vi "SICK Only.vi"() -> ()   [LabVIEW 2009]
uses:
  FPGA/SICK VI's/SICK Reader States.ctl
  Init State.ctl
  <vilib>/LabVIEW Targets/FPGA/cRIO/shared/nicrio_ModuleControls/nicrio_cRIO-9871_FlowControlEnum.ctl
  <vilib>/LabVIEW Targets/FPGA/cRIO/shared/nicrio_ModuleControls/nicrio_cRIO-9871_ParityEnum.ctl
  <vilib>/LabVIEW Targets/FPGA/cRIO/shared/nicrio_ModuleControls/nicrio_cRIO-9871_StopBitsEnum.ctl
  <vilib>/LabVIEW Targets/FPGA/cRIO/shared/nicrio_ModuleControls/nicrio_cRIO-9871_DataBitsEnum.ctl
  <vilib>/LabVIEW Targets/FPGA/cRIO/shared/nicrio_ModuleControls/nicrio_cRIO-9871_BaudRateEnum.ctl
  <vilib>/eio/EIOPropertyNode/EIOPropertyNode.xnode
  <vilib>/rvi/eio/nirviEIOPropertyImplementation/nirviEIOPropertyImplementation.xnode
  <vilib>/rvi/eio/common/nirviEmuTemplatePropertySet_errors.vi
  <vilib>/eio/EIOMethodNode/EIOMethodNode.xnode
  <vilib>/rvi/eio/nirviEIOMethodImplementation/nirviEIOMethodImplementation.xnode
  <vilib>/rvi/eio/common/nirviEmuTemplateMethod_errors.vi
  <vilib>/rvi/eio/common/nirviEmuClasses.ctl
  <vilib>/rvi/DataTransferAndStorage/Container/XNode/niFpgaContainer.xnode
  <vilib>/rvi/interface/RandomDataEmulation/niFpgaRandomDataHandleErrors.vi
  <vilib>/rvi/interface/RandomDataEmulation/nirviRandomDataFPGAFIFO.vi
  <vilib>/rvi/DataTransferAndStorage/Container/Common/niFpgaContainerMethod.ctl
  <vilib>/rvi/DataTransferAndStorage/Container/Common/niFpgaTransferTypeControl.ctl
  <vilib>/rvi/Memory/Memory_Emulation/nirvimemoryEmulationManagerCache_GetValue.vi
  <vilib>/rvi/Memory/Memory_Emulation/nirvimemoryEmulationManagerCache_InsertValue.vi
  <vilib>/rvi/FIFO/Fifo_Resource/nirvififoUniquifyingName.vi
  <vilib>/Utility/error.llb/Clear Errors.vi
  <vilib>/rvi/Memory/Memory_Emulation/nirvimemoryEmulationManagerCache_SetValue.vi
  <vilib>/rvi/eio/common/nirviEmuTemplatePropertyGet_errors.vi
panel:
  out "Responses Timeout":bool
  in  "Correct Response Timeout (ms)":i32=200
  out "SICK Init State":u8
  out "SICK Reader States":T1
  in  "EN mask overflow bytes":bool
  in  "En overflow replacement":bool
  out "Read Period":u32
  out "Tick count":u32
  out "Read data error":errorcluster
  in  "Read/Write Timeout (ms)":i32
  in  "Bytes at Port Timeout (us)":i32
  in  "Overflow Reading":u16
  out "No Data (timeout)":bool
  out "Initialization error":errorcluster
  out "RT commands timeout":bool
  out "Pre-initialization error":errorcluster
  out "Initialization success":bool
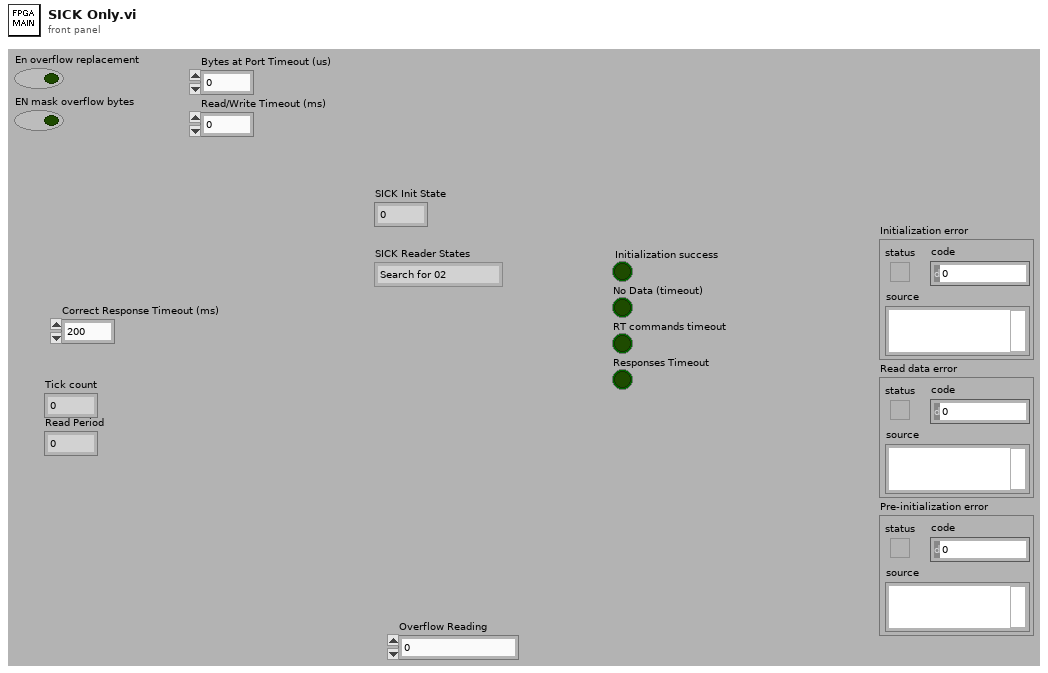
[diagram p1: front panel]
types:
  T1 = typedef "SICK Reader States.ctl" = enum16{"Search for 02", "Search for Header", "Read Data"}
  T2 = typedef "Init State.ctl" = u8
  T3 = typedef "nicrio_cRIO-9871_FlowControlEnum.ctl" = enum8{"None", "Software (XON / XOFF)", "Hardware (RTS / CTS)"}
  T4 = typedef "nicrio_cRIO-9871_ParityEnum.ctl" = enum8{"None", "Odd", "Even", "Mark", "Space"}
  T5 = typedef "nicrio_cRIO-9871_StopBitsEnum.ctl" = enum8{"1", "1.5", "2"}
  T6 = typedef "nicrio_cRIO-9871_DataBitsEnum.ctl" = enum8{"5", "6", "7", "8"}
  T7 = typedef "nicrio_cRIO-9871_BaudRateEnum.ctl" = enum16{"75 bps", "110 bps", "134 bps", "150 bps", "300 bps", "600 bps", "1200 bps", "1800 bps", "2400 bps", "4800 bps", "7200 bps", "9600 bps", "14.4 kbps", "19.2 kbps", "28.8 kbps", "38.4 kbps", "57.6 kbps", "115.2 kbps", "230.4 kbps", "460.8 kbps", "921.6 kbps"}
  T8 = typedef "nirviEmuClasses.ctl" = enum16{"IO Read", "IO Write", "Method", "Property Read", "Property Write"}
  T9 = typedef "niFpgaContainerMethod.ctl" = enum16{"Write", "Read", "Clear", "Get Number of Elements to Write", "Get Number of Elements to Read", "Enable", "Disable", "Flush and Disable", "Get Stream State"}
  T10 = typedef "niFpgaTransferTypeControl.ctl" = enum16{"Target-Scoped", "Host to Target - DMA", "Target to Host - DMA", "Peer to Peer Reader", "Peer to Peer Writer", "Bidirectional"}
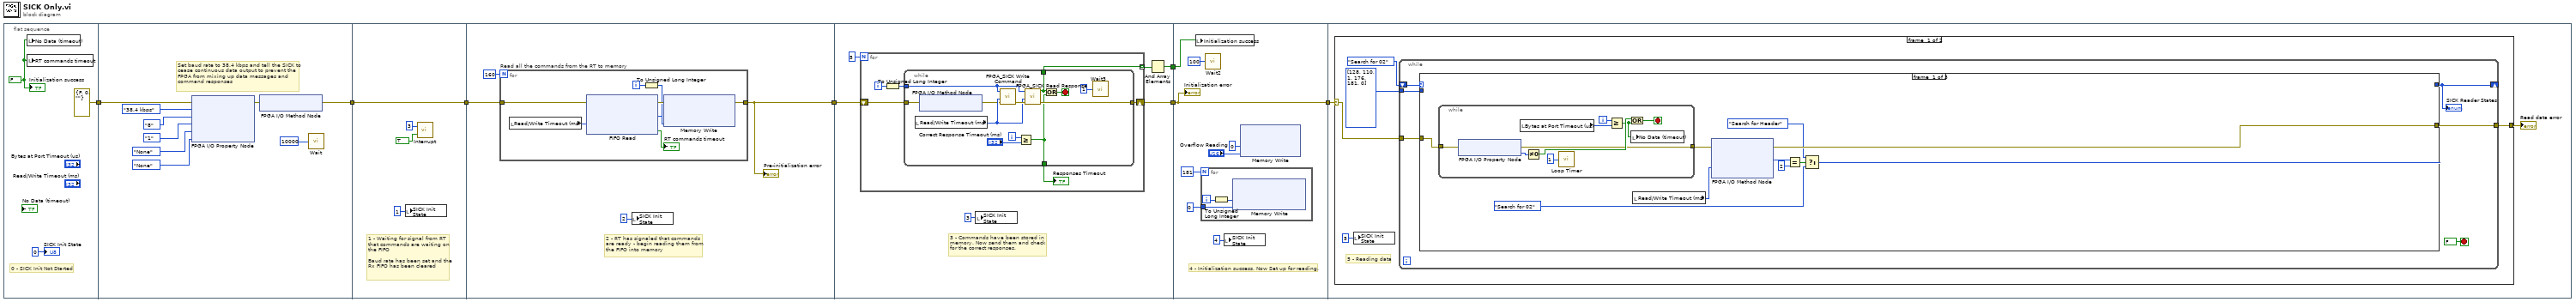
[diagram p0: block diagram]
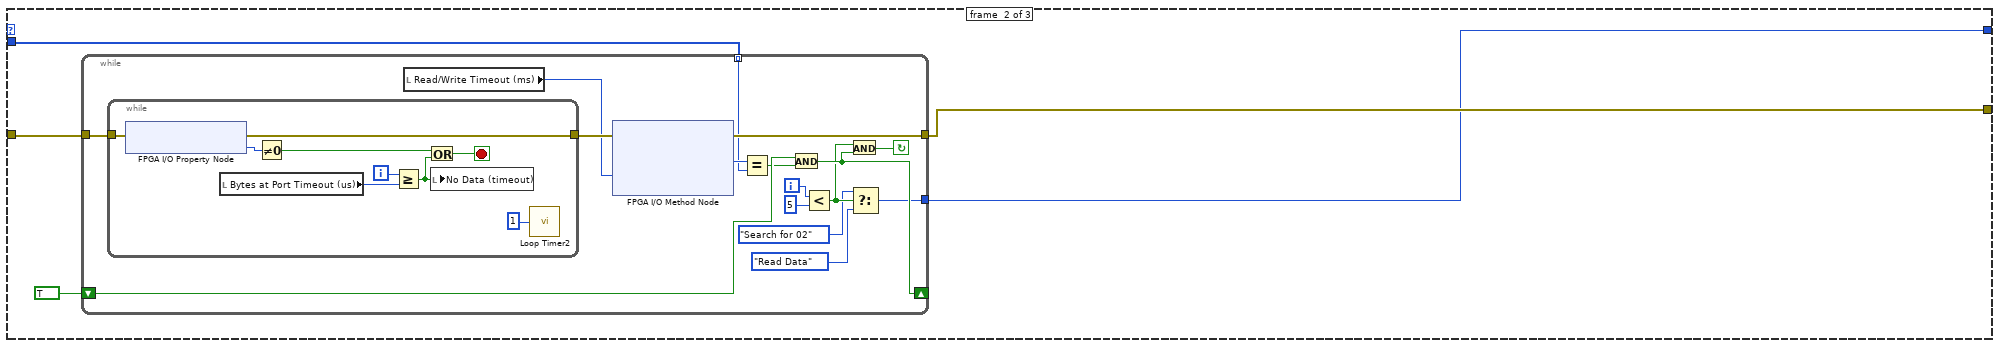
[diagram p2: hidden frame]
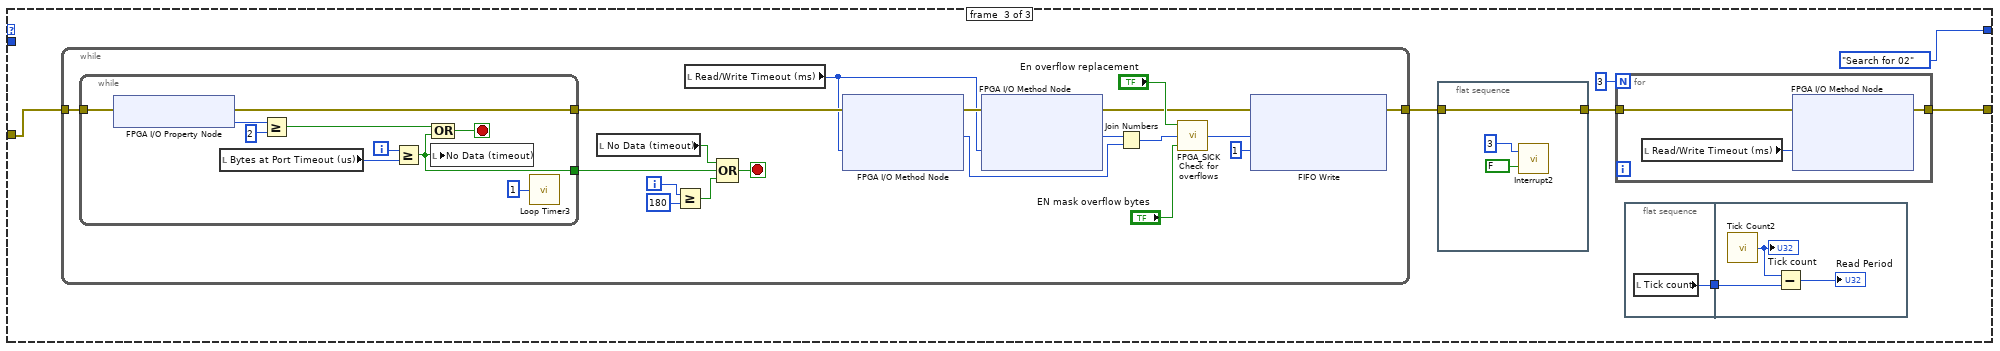
[diagram p3: hidden frame]
diagram:
  n1 = flat-sequence {
    tunnel: [errorcluster {"status"=FALSE, "code"=0, "source"=""} ("error out")] -> w6
    tunnel: w6 -> [w12]
    tunnel: [w11] -> w5
    tunnel: w5 -> [w78]
    tunnel: [w78] -> w4
    tunnel: w4 -> [w82]
    tunnel: [w80] -> w2
    tunnel: [w253] -> w3
    tunnel: w2 -> [w256]
    tunnel: [w252] -> w1
    tunnel: w3 -> [w287]
    tunnel: [w287] -> w7
    tunnel: w1 -> [w286]
    tunnel: w7 -> [w551]
    frame #0 {
      w10 = FALSE ("Initialization complete")
      # "0 - SICK Init Not Started"
      n2 = local write "No Data (timeout)"(w10) -> ()
      n3 = local write "RT commands timeout"(w10) -> ()
      "Initialization success" <- w10
      "SICK Init State" <- T2 0 ("SICK Init State")
    }
    frame #1 {
      # "Set baud rate to 38.4 kbps and tell the SICK to \ncease continuous data output to prevent the \nFPGA from mixing up data messages and \ncommand responses"
      n4 = xnode "FPGA I/O Property Node"("error in"=w12, "Baud Rate"=nicrio_cRIO-9871_BaudRateEnum."38.4 kbps", "Data Bits"=nicrio_cRIO-9871_DataBitsEnum."8", "Stop Bits"=nicrio_cRIO-9871_StopBitsEnum."1", "Parity"=nicrio_cRIO-9871_ParityEnum."None", "Flow Control"=nicrio_cRIO-9871_FlowControlEnum."None") -> ("error out"=w14:errorcluster)  [unwired: 1 in, 1 out]
      n5 = xnode "FPGA I/O Method Node"("error in"=w14) -> ("error out"=w11:errorcluster)  [unwired: 1 in, 1 out]
      n6 = call "Wait"("Count(uSec)"=u32 10000 ("Set new baud rate wait (usec)")) -> ()  [unwired: 1 out]
    }
    frame #2 {
      # "1 - Waiting for signal from RT\nthat commands are waiting on\nthe FIFO\n\nBaud rate has been set and the\nRx FIFO has been cleared"
      n7 = local write "SICK Init State"(T2 1 ("SICK Init State")) -> ()
      n8 = call "Interrupt"("Wait Until Cleared"=TRUE, "IRQ Number"=u8 3) -> ()  [unwired: 1 out]
    }
    frame #3 {
      # "2 - RT has signaled that commands\nare ready - begin reading them from\nthe FIFO into memory"
      n9 = for "Read all the commands from the RT to memory" {
        N: 160 -> [_]
        tunnel: [w89] -> w80
        tunnel: w82 -> [w84]
        i -> [w86]
        n10 = local read "Read/Write Timeout (ms)"() -> (w88:i32)
        n11 = xnode ("FIFO Read")("Timeout"=w88, "error in (no error)"=w84) -> ("Element"=w91:u8, "Timed Out?"=→"RT commands timeout":bool, "error out"=w90:errorcluster)  [unwired: 1 in, 1 out]
        n12 = To Unsigned Long Integer(number=w86) -> (unsigned 32bit integer=w85:u32)
        n13 = xnode ("Memory Write")("Address"=w85, "Data"=w91, "error in (no error)"=w90) -> ("error out"=w89:errorcluster)  [unwired: 1 in, 1 out]
      }
      "Pre-initialization error" <- w80
      n14 = local write "SICK Init State"(T2 2 ("SICK Init State")) -> ()
    }
    frame #4 {
      # "3 - Commands have been stored in\nmemory. Now send them and check\nfor the correct responses."
      n15 = for {
        N: 5 -> [_]
        shift-right: [w261] -> w253
        shift-left: w256 -> [w262]
        tunnel: [w258] -> w254 mode=indexing
        i -> [w260]
        n16 = To Unsigned Long Integer(number=w260) -> (unsigned 32bit integer=w259:u32)
        n17 = while {
          tunnel: w262 -> [w265]
          tunnel: [w274] -> w261
          tunnel: w259 -> [w271]
          tunnel: [w270] -> w258
          tunnel: [w263] -> w257
          i -> [w268]
          stop <- w266 stop-if-true
          n18 = local read "Read/Write Timeout (ms)"() -> (w272:i32)
          n19 = xnode "FPGA I/O Method Node"("error in"=w265) -> ("error out"=w264:errorcluster)  [unwired: 1 in, 1 out]
          n20 = call "FPGA_SICK Write Command.vi"("error in (no error)"=w264, "Read/Write Timeout (ms)"=w272, "Command index"=w271) -> ("error out"=w273:errorcluster)  [unwired: 8 out]
          n21 = Greater Or Equal?(x=w268, y="Correct Response Timeout (ms)") -> (x >= y?=w263:bool)
          n22 = call "FPGA_SICK Read Response.vi"("error in (no error)"=w273, "Timeout (ms)"=w272, "Response Index"=w271) -> ("error out"=w274:errorcluster, "Correct Response Read?"=w270:bool)  [unwired: 7 out]
          n23 = Or(x=w270, y=w263) -> (x .or. y?=w266:bool)
          n24 = call "Wait3"("Count(mSec)"=u8 1 ("Count(Ticks)")) -> ()  [unwired: 1 out]
        }
        "Responses Timeout" <- w257
      }
      n25 = local write "SICK Init State"(T2 3 ("SICK Init State")) -> ()
      n26 = And Array Elements(Boolean array=w254) -> (logical AND=w252:bool)
    }
    frame #5 {
      # "4 - Initialization success. Now Set up for reading."
      n27 = local write "Initialization success"(w286) -> ()
      n28 = for {
        N: 181 -> [_]
        tunnel: u16 0 ("Data") -> [w420]
        i -> [w422]
        n29 = To Unsigned Long Integer(number=w422) -> (unsigned 32bit integer=w421:u32)
        n30 = xnode ("Memory Write")("Address"=w421, "Data"=w420) -> ()  [unwired: 1 in, 1 out]
      }
      n31 = call "Wait2"("Count(mSec)"=u8 100 ("Count(Ticks)")) -> ()  [unwired: 1 out]
      n32 = local write "SICK Init State"(T2 4 ("SICK Init State")) -> ()
      n33 = xnode ("Memory Write")("Address"=u32 0, "Data"="Overflow Reading") -> ()  [unwired: 1 in, 1 out]
      "Initialization error" <- w287
    }
    frame #6 {
      n34 = case shown="No Error" w551 {
        selector: w551 -> [w553 w928]
        tunnel: [w554 w928] -> w550
        frame #0 {
          # "5 - Reading data"
          n35 = local write "SICK Init State"(T2 5 ("SICK Init State")) -> ()
          n36 = while {
            tunnel: u8[] [128, 110, 1, 176, 181, 0] -> [w561]
            tunnel: w553 -> [w560]
            shift-right: [w559] -> _
            shift-left: SICK_Reader_States."Search for 02" ("SICK Reader States") -> [w562]
            tunnel: [w558] -> w554
            stop <- FALSE stop-if-true
            n37 = case shown="\"Read Data\"" w562 {
              tunnel: w561 -> [_ w642 _]
              tunnel: w560 -> [w572 w641 w730]
              tunnel: [w570 w640 w727] -> w558
              tunnel: [w563 w638 SICK_Reader_States."Search for 02" ("SICK Reader States")] -> w559
              frame #0 {
                n38 = while {
                  tunnel: [w576] -> w571
                  tunnel: w572 -> [w574]
                  i -> [w578]
                  stop <- w580 stop-if-true
                  n39 = xnode "FPGA I/O Property Node"("error in"=w574) -> ("error out"=w576:errorcluster, "Bytes at Port"=w581:u8)  [unwired: 1 in, 1 out]
                  n40 = local read "Bytes at Port Timeout (us)"() -> (w575:i32)
                  n41 = Not Equal To 0?(x=w581) -> (x != 0?=w579:bool)
                  n42 = call "Loop Timer"("Count(uSec)"=u8 1) -> ()  [unwired: 1 out]
                  n43 = Greater Or Equal?(x=w578, y=w575) -> (x >= y?=w573:bool)
                  n44 = Or(x=w579, y=w573) -> (x .or. y?=w580:bool)
                  n45 = local write "No Data (timeout)"(w573) -> ()
                }
                n46 = local read "Read/Write Timeout (ms)"() -> (w569:i32)
                n47 = xnode "FPGA I/O Method Node"("error in"=w571, "Timeout (ms)"=w569) -> ("error out"=w570:errorcluster, "Data"=w568:u8)  [unwired: 1 in, 2 out]
                n48 = Equal?(x=w568, y=u8 2) -> (x = y?=w566:bool)
                n49 = Select(t=SICK_Reader_States."Search for Header" ("SICK Reader States"), s=w566, f=SICK_Reader_States."Search for 02" ("SICK Reader States")) -> (s? t:f=w563:T1)
              }
              frame #1 {
                n50 = while {
                  tunnel: w642 -> [w654] mode=indexing
                  tunnel: w641 -> [w656]
                  tunnel: [w655] -> w640
                  shift-right: [w650] -> _
                  shift-left: TRUE ("x = y?") -> [w652]
                  tunnel: [w645] -> w638
                  i -> [w649]
                  stop <- w647 continue-if-true
                  n51 = while {
                    tunnel: [w662] -> w657
                    tunnel: w656 -> [w661]
                    i -> [w664]
                    stop <- w666 stop-if-true
                    n52 = xnode "FPGA I/O Property Node"("error in"=w661) -> ("error out"=w662:errorcluster, "Bytes at Port"=w667:u8)  [unwired: 1 in, 1 out]
                    n53 = local read "Bytes at Port Timeout (us)"() -> (w660:i32)
                    n54 = Not Equal To 0?(x=w667) -> (x != 0?=w665:bool)
                    n55 = Greater Or Equal?(x=w664, y=w660) -> (x >= y?=w659:bool)
                    n56 = Or(x=w665, y=w659) -> (x .or. y?=w666:bool)
                    n57 = local write "No Data (timeout)"(w659) -> ()
                    n58 = call "Loop Timer2"("Count(uSec)"=u8 1) -> ()  [unwired: 1 out]
                  }
                  n59 = local read "Read/Write Timeout (ms)"() -> (w653:i32)
                  n60 = xnode "FPGA I/O Method Node"("error in"=w657, "Timeout (ms)"=w653) -> ("error out"=w655:errorcluster, "Data"=w658:u8)  [unwired: 1 in, 2 out]
                  n61 = Equal?(x=w658, y=w654) -> (x = y?=w651:bool)
                  n62 = And(x=w652, y=w651) -> (x .and. y?=w650:bool)
                  n63 = Less?(x=w649, y=5) -> (x < y?=w646:bool)
                  n64 = And(x=w646, y=w650) -> (x .and. y?=w647:bool)
                  n65 = Select(t=SICK_Reader_States."Search for 02" ("SICK Reader States"), s=w646, f=SICK_Reader_States."Read Data" ("SICK Reader States")) -> (s? t:f=w645:T1)
                }
              }
              frame #2 {
                n66 = while {
                  tunnel: w730 -> [w755]
                  tunnel: [w742] -> w724
                  i -> [w746]
                  stop <- w748 stop-if-true
                  n67 = while {
                    tunnel: [w826] -> w756
                    tunnel: w755 -> [w825]
                    tunnel: [w822] -> w740
                    i -> [w828]
                    stop <- w830 stop-if-true
                    n68 = xnode "FPGA I/O Property Node"("error in"=w825) -> ("error out"=w826:errorcluster, "Bytes at Port"=w831:u8)  [unwired: 1 in, 1 out]
                    n69 = local read "Bytes at Port Timeout (us)"() -> (w824:i32)
                    n70 = Greater Or Equal?(x=w831, y=u8 2 ("x")) -> (x >= y?=w829:bool)
                    n71 = Greater Or Equal?(x=w828, y=w824) -> (x >= y?=w822:bool)
                    n72 = local write "No Data (timeout)"(w822) -> ()
                    n73 = Compound Arithmetic op=OR(w829, w822) -> (w830:bool)
                    n74 = call "Loop Timer3"("Count(uSec)"=u8 1) -> ()  [unwired: 1 out]
                  }
                  n75 = local read "No Data (timeout)"() -> (w741:bool)
                  n76 = Greater Or Equal?(x=w746, y=180) -> (x >= y?=w749:bool)
                  n77 = local read "Read/Write Timeout (ms)"() -> (w747:i32)
                  n78 = Compound Arithmetic op=OR(w741, w740, w749) -> (w748:bool)
                  n79 = xnode "FPGA I/O Method Node"("error in"=w756, "Timeout (ms)"=w747) -> ("error out"=w754:errorcluster, "Data"=w752:u8)  [unwired: 1 in, 2 out]
                  n80 = xnode "FPGA I/O Method Node"("error in"=w754, "Timeout (ms)"=w747) -> ("error out"=w743:errorcluster, "Data"=w753:u8)  [unwired: 1 in, 2 out]
                  n81 = Join Numbers(hi=w753, lo=w752) -> ((hi.lo)=w751:u16)
                  n82 = call "FPGA_SICK Check for overflows.vi"("EN mask overflow bytes"="EN mask overflow bytes", "Data chunk in"=w751, "En overflow replacement"="En overflow replacement") -> ("Data chunk out"=w739:u16)
                  n83 = xnode ("FIFO Write")("Element"=w739, "Timeout"=1, "error in (no error)"=w743) -> ("error out"=w742:errorcluster)  [unwired: 1 in, 2 out]
                }
                n84 = flat-sequence {
                  tunnel: [w733] -> w725
                  tunnel: w724 -> [w733]
                  frame #0 {
                    n85 = call "Interrupt2"("Wait Until Cleared"=FALSE, "IRQ Number"=u8 3 ("SICK IRQ")) -> ()  [unwired: 1 out]
                  }
                }
                n86 = for {
                  N: 3 -> [_]
                  tunnel: [w890] -> w727
                  tunnel: w725 -> [w888]
                  n87 = local read "Read/Write Timeout (ms)"() -> (w889:i32)
                  n88 = xnode "FPGA I/O Method Node"("error in"=w888, "Timeout (ms)"=w889) -> ("error out"=w890:errorcluster)  [unwired: 1 in, 3 out]
                }
                n89 = flat-sequence {
                  tunnel: [w734] -> w726
                  tunnel: w726 -> [w737]
                  frame #0 {
                    n90 = local read "Tick count"() -> (w734:u32)
                  }
                  frame #1 {
                    n91 = call "Tick Count2"() -> ("Tick Count(uSec)"=w735:u32)
                    "Tick count" <- w735
                    n92 = Subtract(x=w735, y=w737) -> (x-y=→"Read Period":u32)
                  }
                }
              }
            }
            "SICK Reader States" <- w559
          }
        }
        frame #1 {
        }
      }
      "Read data error" <- w550
    }
  }
